vi "gVar_ECa3.vi"() -> ()   [LabVIEW 2020]
panel:
  out "ECa3":dbl
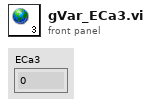
[diagram p1: front panel]
diagram:
